vi "AcquireIMAQImage.vi"(5 "ImagePath":path, 6 "ImageName":string="NewImage", 7 "SaveToDisk?":bool, 8 "error in":errorcluster, 11 "webcam image in":cluster{"image":u8[], "width":i32, "height":i32}) -> (0 "error out":errorcluster, 3 "ImageOut":T1)   [LabVIEW 2013]
doc: "Gets an image from the webcam and converts it to an IMAQ format. The default inputs should be sufficient. Use SaveToDisk? if testing with Vision Assistant is needed."
uses:
  <vilib>/vision/Image Controls.llb/IMAQ Image.ctl
  Lib/Webcam/Webcam Typedefs.llb/Webcam depth.ctl
panel:
  out "Camera Image":T1(plugin-control)
  out "Image":picture
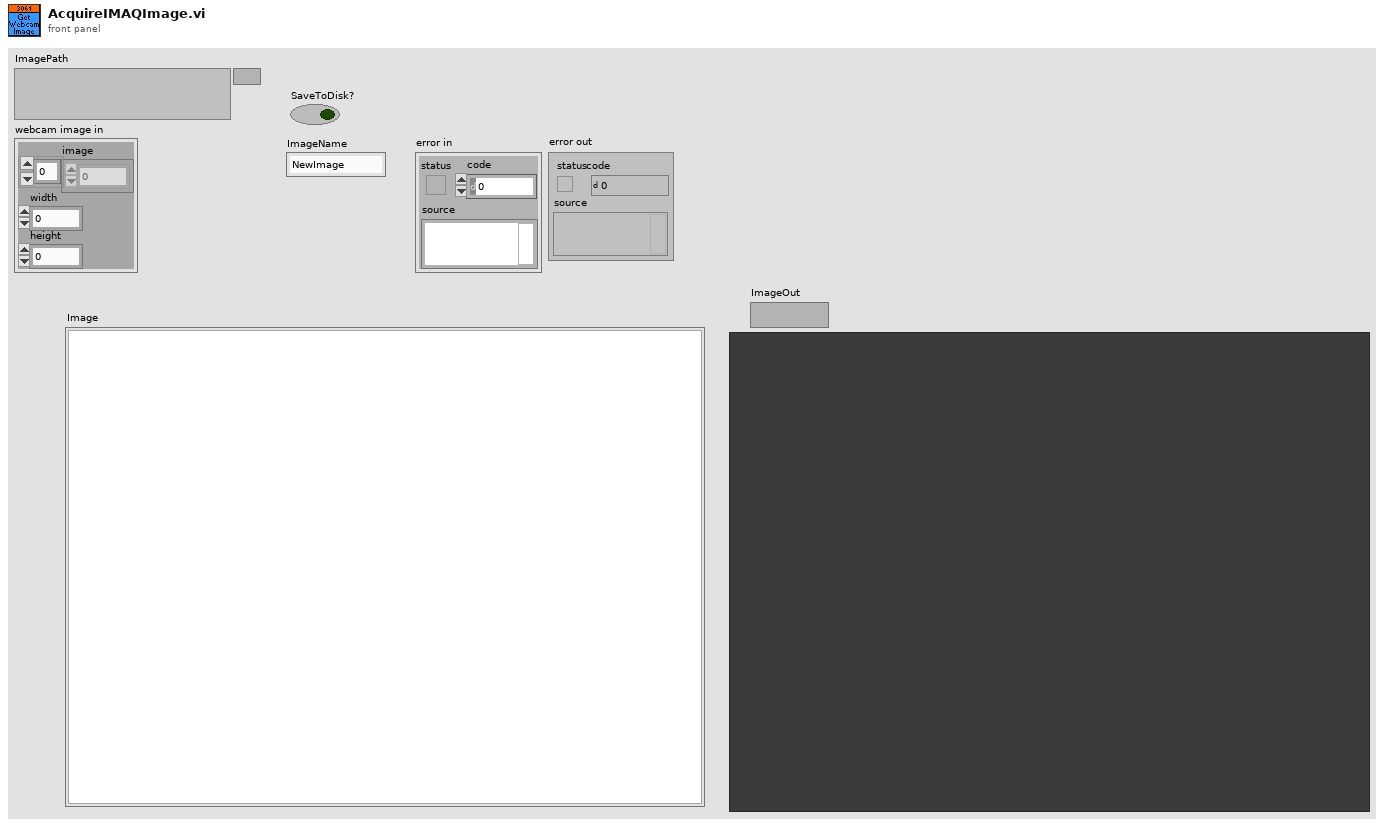
[diagram p1: front panel]
types:
  T1 = typedef "IMAQ Image.ctl" = refnum<image>
  T2 = typedef "Image Type" = u32
  T3 = typedef "Webcam depth.ctl" = enum16{"24-bit", "8-bit"}
  T4 = typedef "Webcam rect.ctl" = cluster{"left":i16, "top":i16, "right":i16, "bottom":i16}
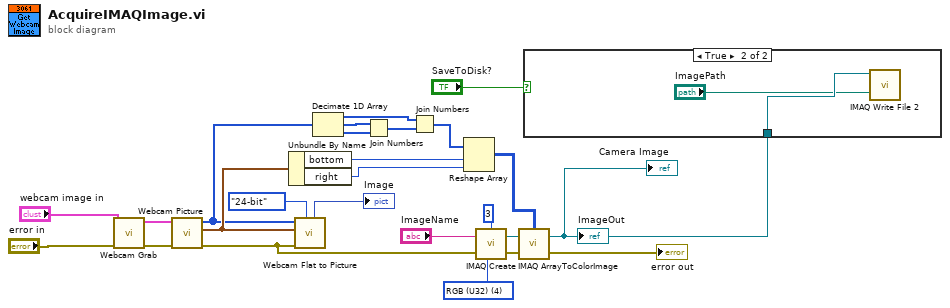
[diagram p0: block diagram]
diagram:
  w11 = T2 4 items=["Grayscale (U8)", "Grayscale (I16)", "Grayscale (SGL)", "Complex (CSG)", "RGB (U32)", "HSL (U32)", "RGB (U64)", "Grayscale (U16)"] ("Image Type")
  n1 = call "Webcam Grab.vi"("error in"="error in", "webcam image in"="webcam image in") -> ("error out"=w6:errorcluster, "webcam image out"=w7:cluster{"image":u8[], "width":i32, "height":i32})  [unwired: 7 in]
  n2 = call "Webcam Picture.vi"("error in"=w6, "webcam image in"=w7) -> ("error out"=w3:errorcluster, "rect"=w5:T4, "flat RGB image"=w4:u8[])  [unwired: 6 in, 1 out]
  n3 = Unbundle By Name(w5) -> ("bottom"=w15:i16, "right"=w14:i16)
  n4 = call "Webcam Flat to Picture.vi"("depth (8)"=Webcam_depth."24-bit", "error in"=w3, "rect in"=w5, "flat image in"=w4) -> ("picture"=→"Image":picture)  [unwired: 3 in, 3 out]
  n5 = Decimate 1D Array(w4) -> (w20:u8[], w23:u8[], w22:u8[])
  n6 = Join Numbers(hi=w23, lo=w22) -> ((hi.lo)=w21:u16[])
  n7 = Join Numbers(hi=w20, lo=w21) -> ((hi.lo)=w19:u32[])
  n8 = Reshape Array(w19, w15, w14) -> (w18:u32[][])
  n9 = call "IMAQ Create"("Border Size"=3, "Image Name"="ImageName", "Image Type"=w11, "error in (no error)"=w3) -> ("New Image"=w17:T1, "error out"=w16:errorcluster)  [unwired: 1 in]
  n10 = call "IMAQ ArrayToColorImage"("Image Pixels (U32)"=w18, "Image"=w17, "error in (no error)"=w16) -> ("Image Out"=w9:T1, "error out"=→"error out":errorcluster)  [unwired: 2 in]
  "ImageOut" <- w9
  "Camera Image" <- w9
  n11 = case shown="True" "SaveToDisk?" {
    tunnel: w9 -> [_ w27]
    frame False {
    }
    frame True {
      n12 = call-poly "IMAQ Write File 2"("File Path"="ImagePath", "Image"=w27) -> ()  [unwired: 8 in, 2 out]
    }
  }
